vi "Class Object Destruction.vi"(7 "class labels":T1=enum."Valve Controller", 8 "error in":errorcluster, 11 "classes in":T2) -> (0 "error out":errorcluster, 3 "classes out":T2)   [LabVIEW 2011]
uses:
  Controls/Class Objects.ctl
  Modules/File/Configuration/Configuration.lvclass
  Modules/Hardware/Power Supply/Power Supply.lvclass
  Modules/Hardware/Mass Flow Controller/Mass Flow Controller.lvclass
  Modules/Hardware/PID/PID.lvclass
  Modules/Hardware/Valve Controller/Valve Controller.lvclass
  Modules/Hardware/Multimeter/Multimeter.lvclass
  Modules/Hardware/Vapour Generator/Vapour Generator.lvclass
  Modules/File/TDMS/TDMS.lvclass
  Controls/Class Labels.ctl
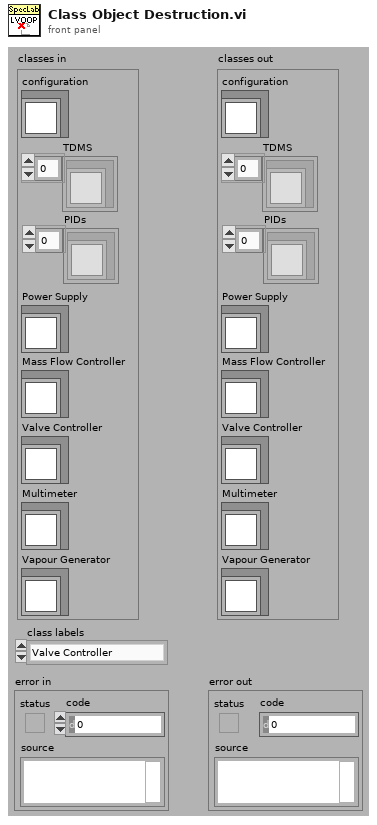
[diagram p1: front panel]
types:
  T1 = typedef "Class Labels.ctl" = enum16{"Configuration", "TDMS", "PID", "Power Supply", "Vapour Generator", "MFC", "NMR", "Valve Controller", "Multimeter"}
  T2 = typedef "Class Objects.ctl" = cluster{"configuration":refnum<class "Configuration.lvclass">, "TDMS":refnum<class "TDMS.lvclass">[], "Power Supply":refnum<class "Power Supply.lvclass">, "Mass Flow Controller":refnum<class "Mass Flow Controller.lvclass">, "Valve Controller":refnum<class "Valve Controller.lvclass">, "Multimeter":refnum<class "Multimeter.lvclass">, "Vapour Generator":refnum<class "Vapour Generator.lvclass">, "PIDs":refnum<class "PID.lvclass">[]}
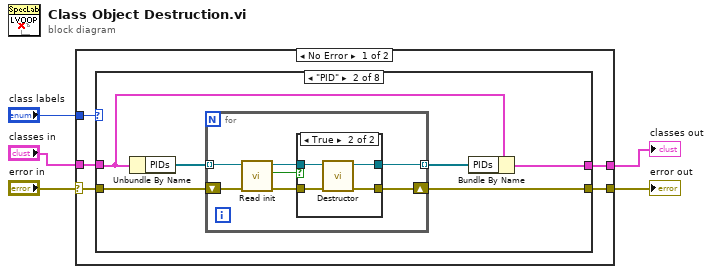
[diagram p0: block diagram]
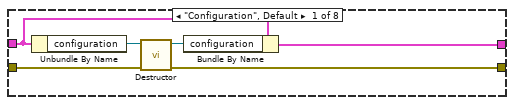
[diagram p2: hidden frame]
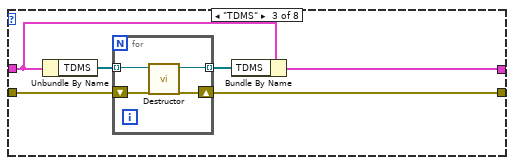
[diagram p4: hidden frame]
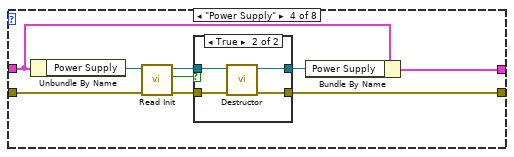
[diagram p5: hidden frame]
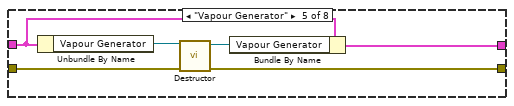
[diagram p7: hidden frame]
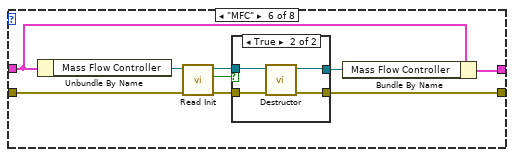
[diagram p8: hidden frame]
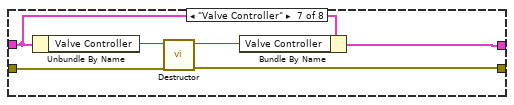
[diagram p10: hidden frame]
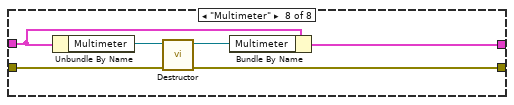
[diagram p11: hidden frame]
diagram:
  n1 = case shown="No Error" "error in" {
    selector: "error in" -> [w10 w95]
    tunnel: [w9 w95] -> w1
    tunnel: "classes in" -> [w8 w94]
    tunnel: "class labels" -> [w7 _]
    tunnel: [w6 w94] -> w2
    frame No Error {
      n2 = case shown="\"PID\"" w7 {
        tunnel: w8 -> [w16 w21 w40 w48 w64 w71 w87 w91]
        tunnel: w10 -> [w13 w20 w37 w54 w66 w74 w85 w90]
        tunnel: [w12 w17 w36 w49 w62 w68 w83 w89] -> w9
        tunnel: [w11 w22 w38 w46 w61 w69 w82 w88] -> w6
        frame "Configuration", Default {
          n3 = Unbundle By Name(w16) -> ("configuration"=w15:refnum<class "Configuration.lvclass">)
          n4 = call-dynamic "Destructor.vi"("error in (no error)"=w13, "Configuration in"=w15) -> ("error out"=w12:errorcluster, "Configuration out"=w14:refnum<class "Configuration.lvclass">)  [unwired: 8 in]
          n5 = Bundle By Name(cluster=w16, "configuration"=w14) -> (w11:T2)
        }
        frame "PID" {
          n6 = Unbundle By Name(w21) -> ("PIDs"=w19:refnum<class "PID.lvclass">[])
          n7 = for {
            tunnel: w19 -> [w25] mode=indexing
            tunnel: [w24] -> w18 mode=indexing
            shift-right: [w23] -> w17
            shift-left: w20 -> [w29]
            n8 = call-dynamic "Read init.vi"("error in (no error)"=w29, "Detector in"=w25) -> ("error out"=w26:errorcluster, "init"=w28:bool, "Detector out"=w27:refnum<class "PID.lvclass">)  [unwired: 7 in]
            n9 = case shown="True" w28 {
              tunnel: [w31 w35] -> w24
              tunnel: [w30 w34] -> w23
              tunnel: w27 -> [w31 w33]
              tunnel: w26 -> [w30 w32]
              frame False {
              }
              frame True {
                n10 = call-dynamic "Destructor.vi"("error in"=w32, "Detector in"=w33) -> ("error out"=w34:errorcluster, "Detector out"=w35:refnum<class "PID.lvclass">)  [unwired: 8 in]
              }
            }
          }
          n11 = Bundle By Name(cluster=w21, "PIDs"=w18) -> (w22:T2)
        }
        frame "TDMS" {
          n12 = Unbundle By Name(w40) -> ("TDMS"=w41:refnum<class "TDMS.lvclass">[])
          n13 = for {
            tunnel: w41 -> [w45] mode=indexing
            tunnel: [w44] -> w39 mode=indexing
            shift-right: [w42] -> w36
            shift-left: w37 -> [w43]
            n14 = call-dynamic "Destructor.vi"("error in"=w43, "TDMS in"=w45) -> ("error out"=w42:errorcluster, "TDMS out"=w44:refnum<class "TDMS.lvclass">)  [unwired: 8 in]
          }
          n15 = Bundle By Name(cluster=w40, "TDMS"=w39) -> (w38:T2)
        }
        frame "Power Supply" {
          n16 = Unbundle By Name(w48) -> ("Power Supply"=w53:refnum<class "Power Supply.lvclass">)
          n17 = call-dynamic "Read Init.vi"("error in (no error)"=w54, "Power Supply in"=w53) -> ("error out"=w51:errorcluster, "Init"=w50:bool, "Power Supply out"=w52:refnum<class "Power Supply.lvclass">)  [unwired: 7 in]
          n18 = case shown="True" w50 {
            tunnel: w52 -> [w56 w60]
            tunnel: w51 -> [w55 w59]
            tunnel: [w56 w58] -> w47
            tunnel: [w55 w57] -> w49
            frame False {
            }
            frame True {
              n19 = call-dynamic "Destructor.vi"("error in (no error)"=w59, "Power Supply in"=w60) -> ("error out"=w57:errorcluster, "Power Supply out"=w58:refnum<class "Power Supply.lvclass">)  [unwired: 8 in]
            }
          }
          n20 = Bundle By Name(cluster=w48, "Power Supply"=w47) -> (w46:T2)
        }
        frame "Vapour Generator" {
          n21 = Unbundle By Name(w64) -> ("Vapour Generator"=w65:refnum<class "Vapour Generator.lvclass">)
          n22 = call-dynamic "Destructor.vi"("error in (no error)"=w66, "Vapour Generator in"=w65) -> ("error out"=w62:errorcluster, "Vapour Generator out"=w63:refnum<class "Vapour Generator.lvclass">)  [unwired: 8 in]
          n23 = Bundle By Name(cluster=w64, "Vapour Generator"=w63) -> (w61:T2)
        }
        frame "MFC" {
          n24 = Unbundle By Name(w71) -> ("Mass Flow Controller"=w75:refnum<class "Mass Flow Controller.lvclass">)
          n25 = call-dynamic "Read Init.vi"("error in (no error)"=w74, "Mass Flow Controller in"=w75) -> ("error out"=w73:errorcluster, "Init"=w67:bool, "Mass Flow Controller out"=w72:refnum<class "Mass Flow Controller.lvclass">)  [unwired: 7 in]
          n26 = case shown="True" w67 {
            tunnel: w72 -> [w77 w81]
            tunnel: w73 -> [w76 w80]
            tunnel: [w77 w79] -> w70
            tunnel: [w76 w78] -> w68
            frame False {
            }
            frame True {
              n27 = call-dynamic "Destructor.vi"("error in (no error)"=w80, "Mass Flow Controller in"=w81) -> ("error out"=w78:errorcluster, "Mass Flow Controller out"=w79:refnum<class "Mass Flow Controller.lvclass">)  [unwired: 8 in]
            }
          }
          n28 = Bundle By Name(cluster=w71, "Mass Flow Controller"=w70) -> (w69:T2)
        }
        frame "Valve Controller" {
          n29 = Unbundle By Name(w87) -> ("Valve Controller"=w86:refnum<class "Valve Controller.lvclass">)
          n30 = call-dynamic "Destructor.vi"("error in (no error)"=w85, "Valve Controller in"=w86) -> ("error out"=w83:errorcluster, "Valve Controller out"=w84:refnum<class "Valve Controller.lvclass">)  [unwired: 8 in]
          n31 = Bundle By Name(cluster=w87, "Valve Controller"=w84) -> (w82:T2)
        }
        frame "Multimeter" {
          n32 = Unbundle By Name(w91) -> ("Multimeter"=w93:refnum<class "Multimeter.lvclass">)
          n33 = call-dynamic "Destructor.vi"("error in (no error)"=w90, "Multimeter in"=w93) -> ("error out"=w89:errorcluster, "Multimeter out"=w92:refnum<class "Multimeter.lvclass">)  [unwired: 8 in]
          n34 = Bundle By Name(cluster=w91, "Multimeter"=w92) -> (w88:T2)
        }
      }
    }
    frame Error {
    }
  }
  "error out" <- w1
  "classes out" <- w2
